vi "Dashboard Main.vi"() -> ()   [LabVIEW 2016]
uses:
  <vilib>/Rock Robotics/WPI/Dashboard/WPI_DashboardLogging Global.vi
  Robot Code/Common Code/Intake Status Cluster.ctl
  Robot Code/Common Code/Climb Status Cluster.ctl
  Robot Code/Common Code/Dash Display Data.ctl
  Robot Code/Common Code/Intake Commands.ctl
  Robot Code/Common Code/Intake Mode.ctl
  Robot Code/Common Code/Intake Presets.ctl
  Robot Code/Common Code/Dashboard Control Data.ctl
  Robot Code/Common Code/Drivetrain Presets.ctl
panel:
  in  "Rec Mode":enum32{"Stop", "Record", "Playback"}(radio)
  in  "Dashboard Tab":T1(tab)
  in  "DB Camera Config":bool
  out "Mbps LED":bool
  out "Mbps":dbl format="%#.1g"
  out "fps":dbl format="%#.1g"
  out "Camera Image":T2(plugin-control)
  out "Intake Power":dbl
  in  "Intake Presets":T3
  out "Intake Status Cluster":T4
  out "DS TCP":T7
  out "Robot Metrics":T8
  out "Camera Info":cluster{}
  in  "Camera Settings":T9={"Frame Rate"=30, "Compression"=30, "Size"=1} {"Frame Rate" scale=1.0..30.0; "Compression" scale=100.0..-1.0; "Size" items=["640x480", "320x240", "160x120"]}
  in  "TCP":refnum<k5>
  out "Robot IP":string
  in  "Camera Name":string(combo)="No Camera Selection"
  # "HW"
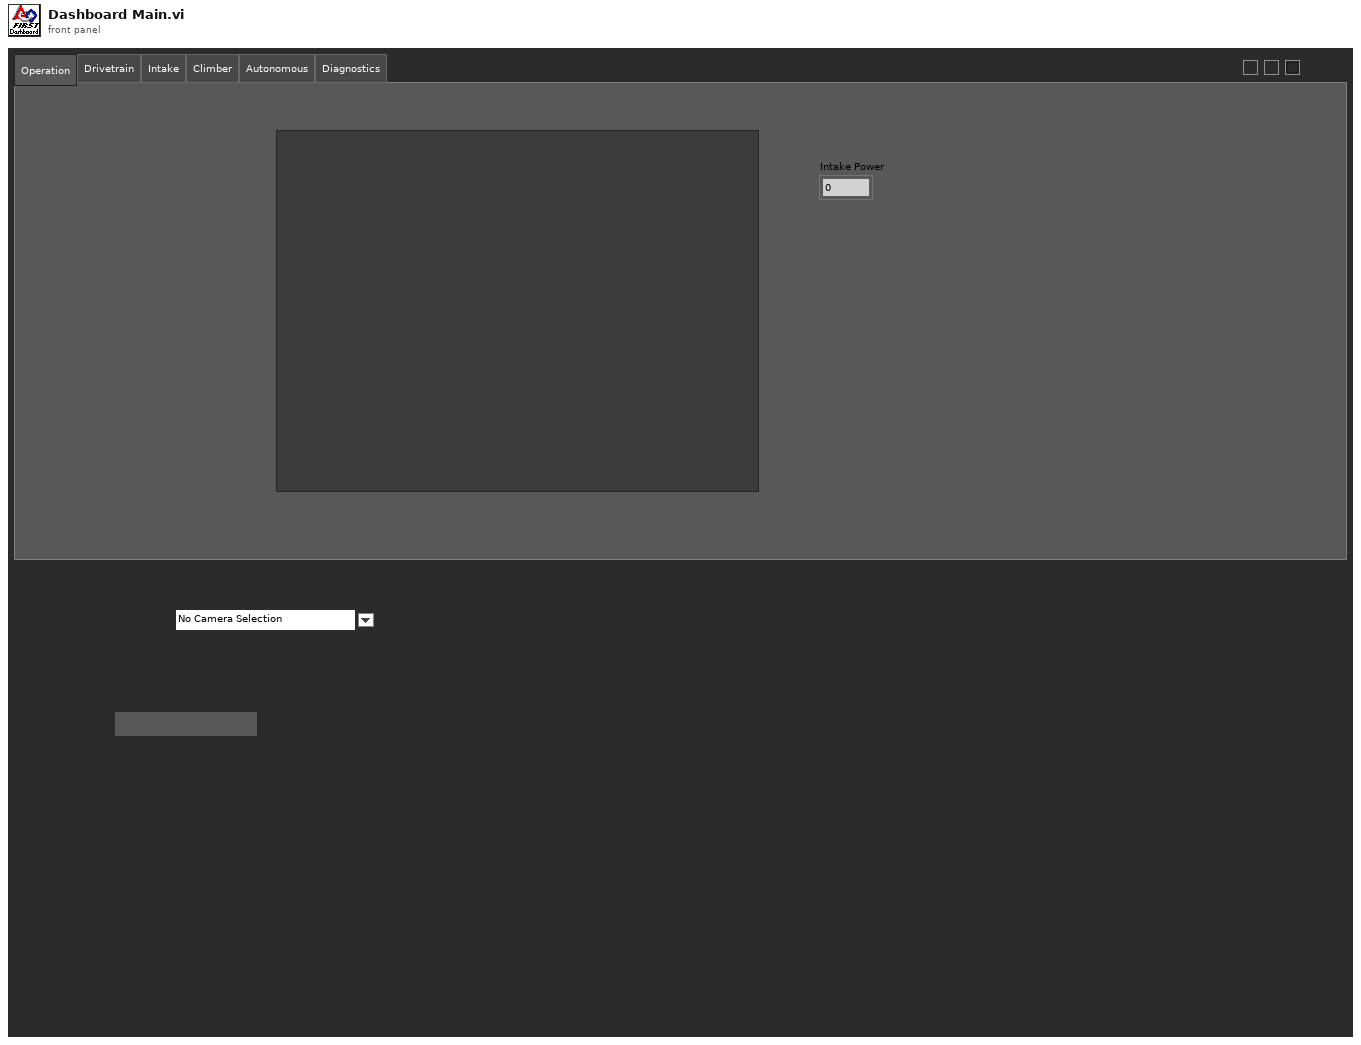
[diagram p1: front panel]
types:
  T1 = enum32{"Operation", "Drivetrain", "Intake", "Climber", "Autonomous", "Diagnostics"}
  T2 = typedef "IMAQ Image.ctl" = refnum<image>
  T3 = typedef "Intake Presets.ctl" = cluster{"Intake Power":dbl, "Outtake Power":dbl}
  T4 = typedef "Intake Status Cluster.ctl" = cluster{"Intake Power":dbl, "Intake Mode":T5, "Intake Command":T6}
  T5 = typedef "Intake Mode.ctl" = enum16{"Manual", "Auto"}
  T6 = typedef "Intake Commands.ctl" = enum16{"Idle", "Intake", "Outtake"}
  T7 = cluster{"Error Strings":string, "Disable Counts":cluster{u16, u16}, "Rail Faults":cluster{u16, u16, u16}, "Robot IP":string, "DB Mode":u8, "Event Info":cluster{"Name":string, "Type":u8, "Number":u16, "Replay":u8}, "Camera Addr":string}
  T8 = cluster{"Storage":cluster{"Disk Free":u64, "RAM Block":u32, "RAM free":u32}, "CPU Utilization":cluster{"CPU % ISR":sgl, "CPU % Time Crit":sgl, "CPU % Timed Str":sgl, "CPU % High":sgl, "CPU % Above":sgl, "CPU % Normal":sgl, "CPU % Low":sgl}, "CAN":cluster{"% Bus Utilization":sgl, "Bus Off Cnt":u32, "TX_FIFO Full Cnt":u32, "Receive Error Cnt":u8, "Transmit Error Cnt":u8}, "HID":cluster{"HID Outputs":u32, "Rumble Low":u16, "Rumble High":u16}[]}
  T9 = cluster{"Frame Rate":i32, "Compression":i32, "Size":u16}
  T10 = cluster{"IDs":cluster{"RPC field ID":u16, "Unique ID":u16}, "String":string}
  T11 = enum32{"Drive", "Basic", "Custom", "Test", "Checklist", "Variables"}
  T12 = typedef "Image Type" = u32
  T13 = typedef "Dashboard Control Data.ctl" = cluster{"Intake Presets":T3, "Drivetrain Presets":T14}
  T14 = typedef "Drivetrain Presets.ctl" = cluster{"Steer PID output":cluster{"output high":dbl, "output low":dbl}, " Steer PID gains":cluster{"proportional gain (Kc)":dbl, "integral time (Ti, min)":dbl, "derivative time (Td, min)":dbl}, "Gyro Tolerance":dbl}
  T15 = typedef "Dash Display Data.ctl" = cluster{"Intake Status Cluster ":T4, "Climb Status Cluster":T16}
  T16 = typedef "Climb Status Cluster.ctl" = cluster{"Power":dbl}
  T17 = cluster{"Status bits":cluster{"Test Mode":bool, "Autonomous":bool, "Enabled":bool, "Code Start":bool, "Brownout":bool, "Reserved 2":bool, "Reserved 3":bool, "E-Stop":bool}, "Code Trace":cluster{"Disabled":bool, "TeleOp":bool, "Auto":bool, "Test":bool}, "Controller Type":enum16{"unknown", "cRIO", "roboRio"}, "Code?":enum16{"unknown", "noCode", "code"}, "Battery V":dbl}
  T18 = cluster{"Control Bits":cluster{"TestMode":bool, "Autonomous":bool, "Enabled":bool, "FMS Present":bool, bool, bool, bool, "E-Stop":bool}, "Team Station ":u8, "Countdown":sgl, "Joystick Values":cluster{"Axes":dbl[], "Buttons":bool[], "POVs":i16[]}[]}
  T19 = enum8{"Tele-Op Disabled", "Tele-Op Enabled", "Auto Disabled", "Auto Enabled", "Test Disabled", "Test Enabled", "Disconnected", "No Code", "E-Stop"}
  T20 = cluster{"Image Size":bool, "Image Type":bool, "Pixel Value":bool, "ROI Information":bool, "Zoom Factor":bool}
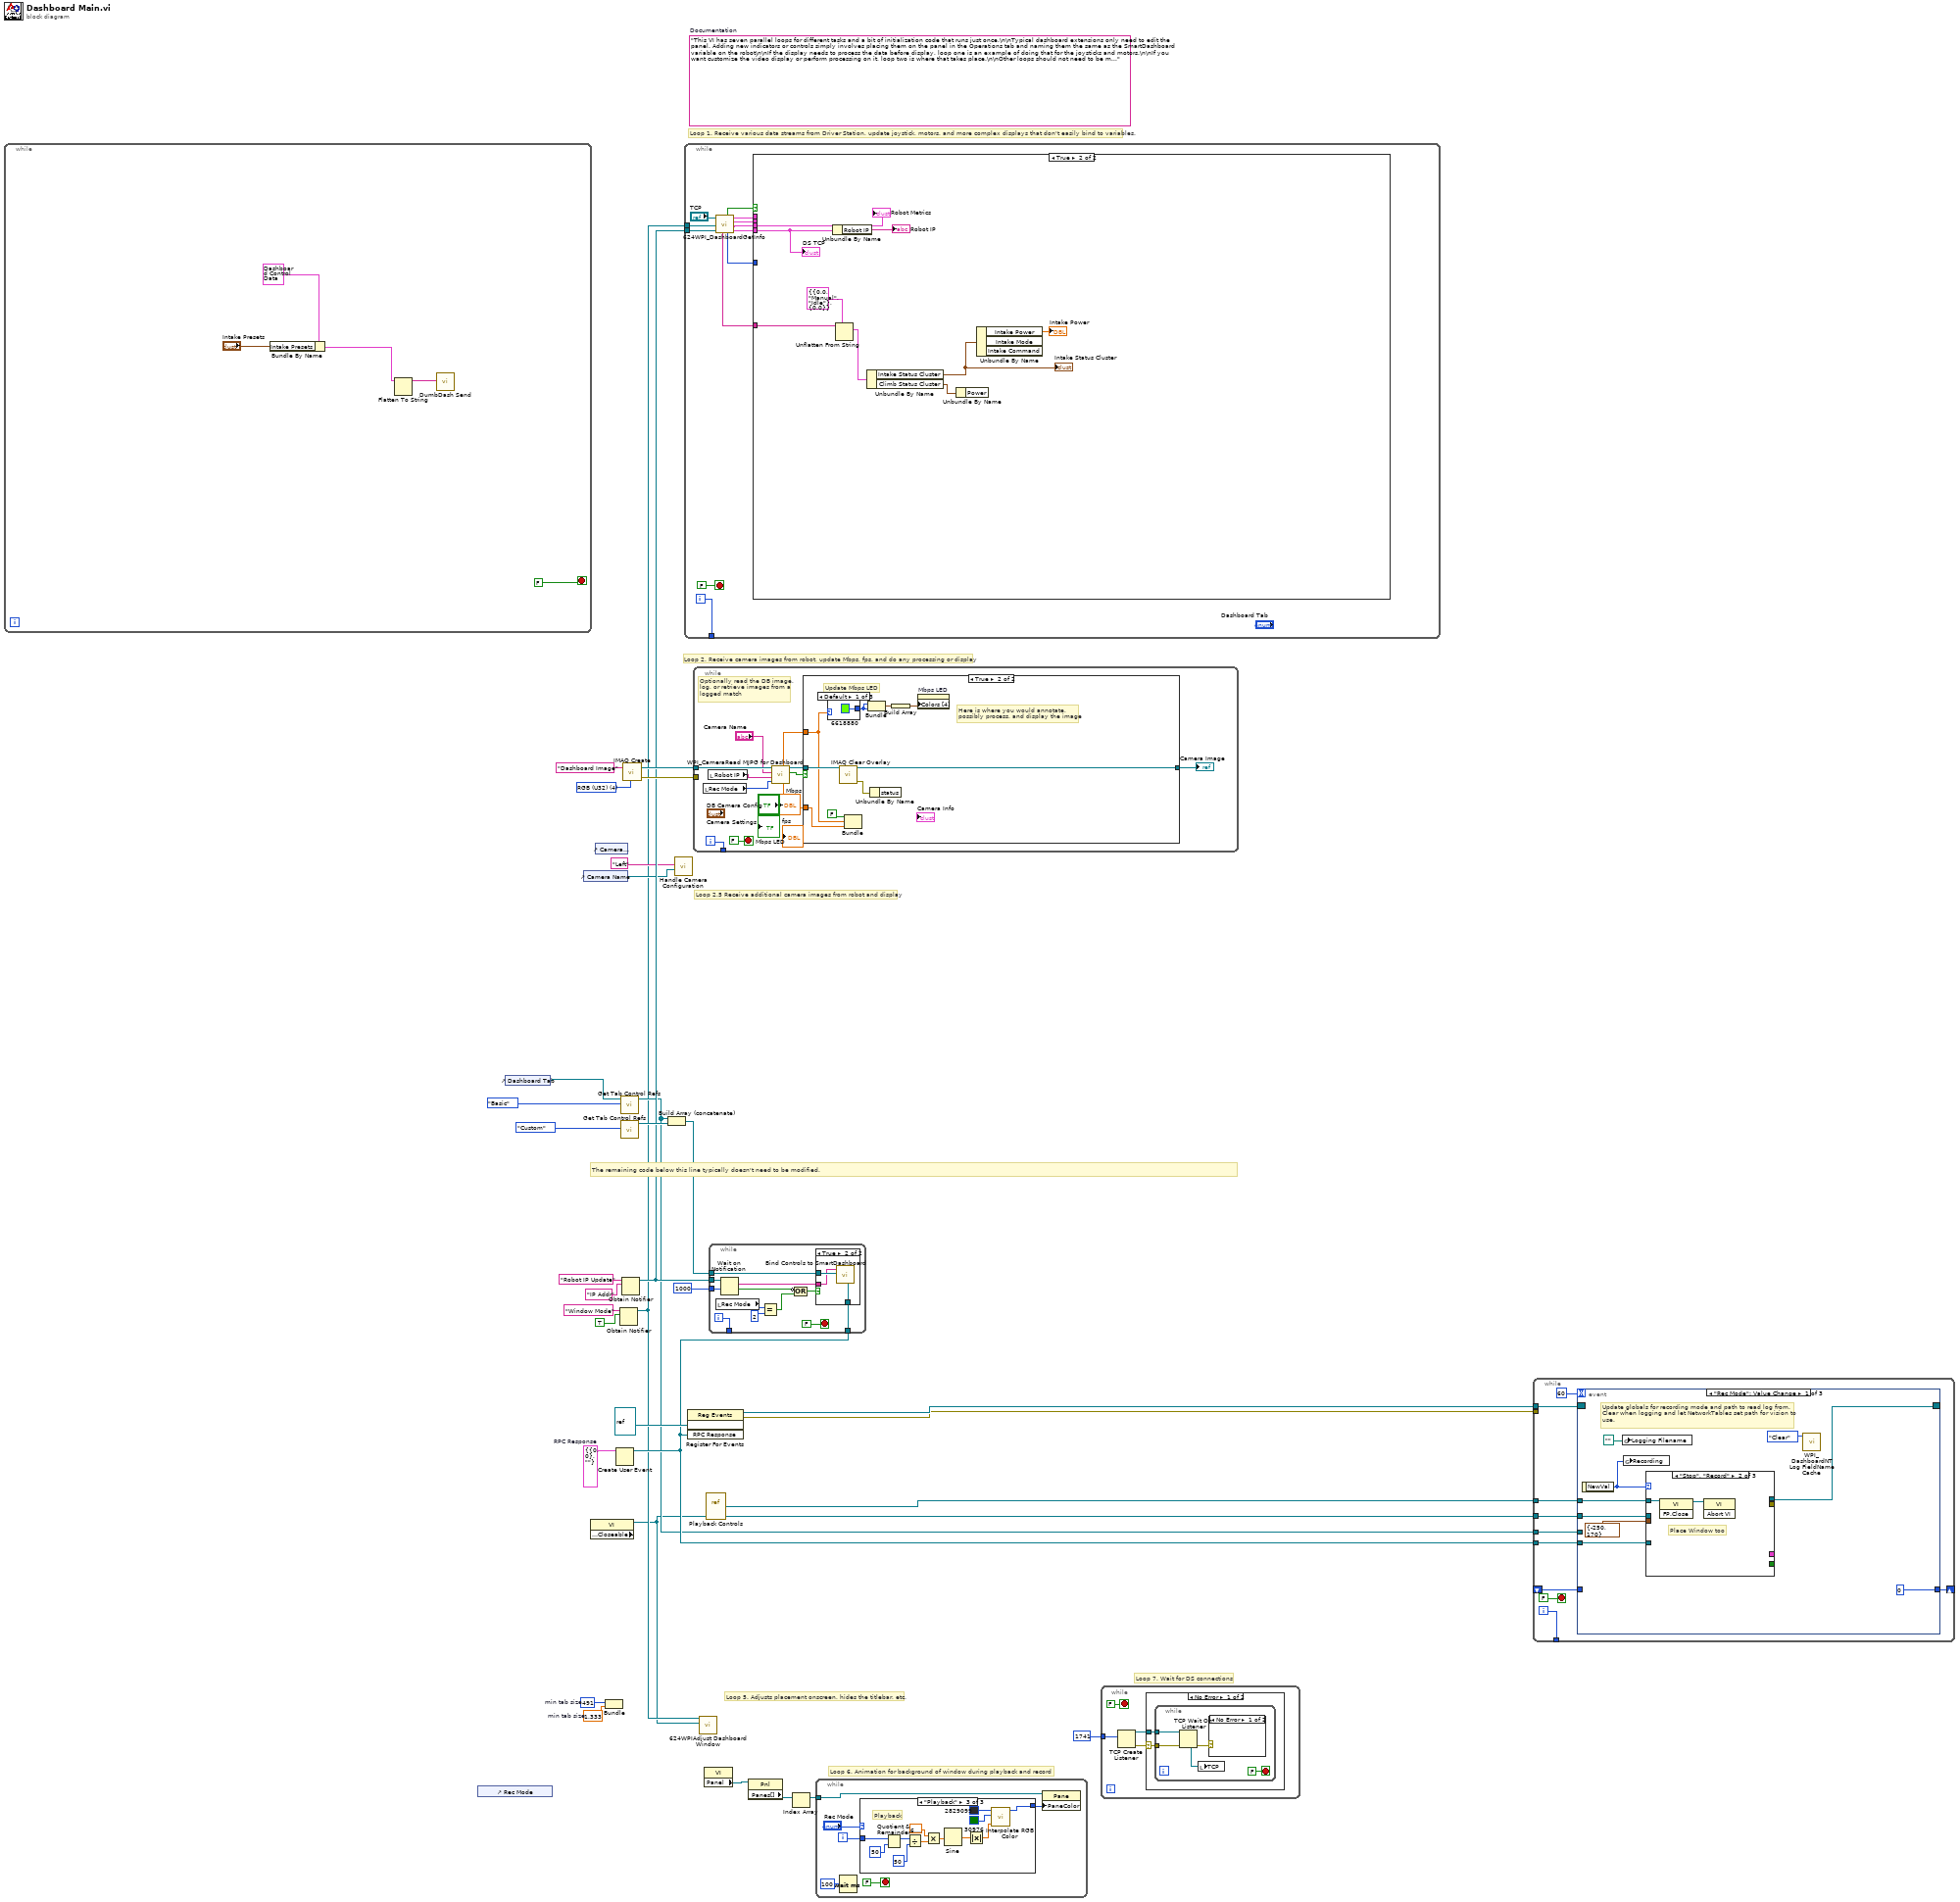
[diagram p0: block diagram]
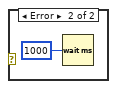
[diagram p2: hidden frame]
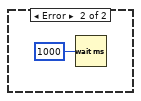
[diagram p3: hidden frame]
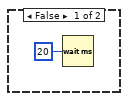
[diagram p4: hidden frame]
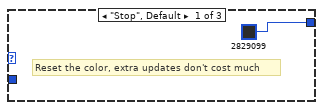
[diagram p5: hidden frame]
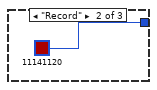
[diagram p6: hidden frame]
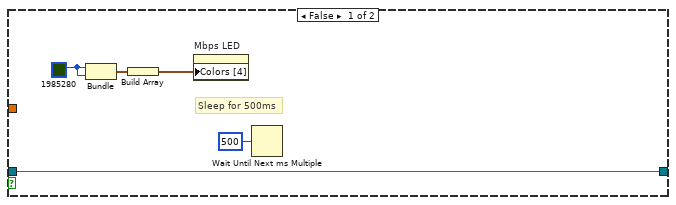
[diagram p8: hidden frame]
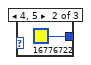
[diagram p9: hidden frame]
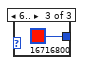
[diagram p10: hidden frame]
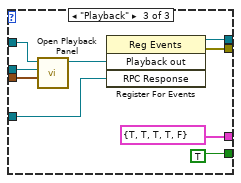
[diagram p12: hidden frame]
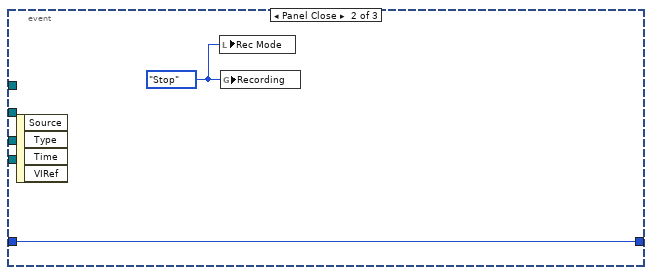
[diagram p13: hidden frame]
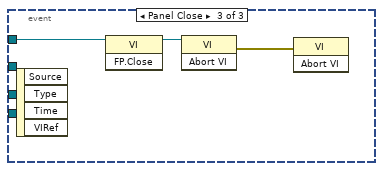
[diagram p14: hidden frame]
diagram:
  w8 = T10 {"IDs"={"RPC field ID"=0, "Unique ID"=0}, "String"=""}  # RPC Response
  w14 = 491  # min tab size
  w13 = 1.333  # min tab size
  (unwired) "This VI has seven parallel loops for different tasks and a bit of initialization code that runs just once.\n\nTypical dashboard extensions only need to edit the panel. Adding new indicators or controls simply involves placing them on the panel in the Operations tab and naming them the same as the SmartDashboard variable on the robot\n\nIf the display needs to process the data before display, loop one is an example of doing that for the joysticks and motors.\n\nIf you want customize the video display or perform processing on it, loop two is where that takes place.\n\nOther loops should not need to be modified. They are pretty standard, and document the task they perform."  # Documentation
  w32 = T12 4 items=["Grayscale (U8)", "Grayscale (I16)", "Grayscale (SGL)", "Complex (CSG)", "RGB (U32)", "HSL (U32)", "RGB (U64)"] ("Image Type")
  # "Loop 2.5 Receive additional camera images from robot and display"
  # "Loop 7. Wait for DS connections"
  # "Loop 6. Animation for background of window during playback and record"
  # "The remaining code below this line typically doesn't need to be modified."
  # "Loop 5. Adjusts placement onscreen, hides the titlebar, etc."
  # "Loop 1. Receive various data streams from Driver Station, update joystick, motors, and more complex displays that don't easily bind to variables."
  # "Loop 2. Receive camera images from robot, update Mbps, fps, and do any processing or display"
  n1 = while {
    stop <- FALSE stop-if-true
    n2 = Bundle By Name(cluster=T13 {"Intake Presets"={"Intake Power"=0.0, "Outtake Power"=0.0}, "Drivetrain Presets"={"Steer PID output"={"output high"=0.0, "output low"=0.0}, " Steer PID gains"={"proportional gain (Kc)"=0.0, "integral time (Ti, min)"=0.0, "derivative time (Td, min)"=0.0}, "Gyro Tolerance"=0.0}} ("Dashboard Packet"), "Intake Presets"="Intake Presets") -> (w34:T13)
    n3 = Flatten To String(anything=w34) -> (data string=w36:string)  [unwired: 3 in, 2 out]
    n4 = call "DumbDash Send.vi"("data string"=w36) -> ()  [unwired: 11 in]
  }
  n5 = control-ref of="Rec Mode"() -> ()  [unwired: 1 out]
  n6 = control-ref of="Dashboard Tab"() -> (w1:refnum<vi>)
  n7 = control-ref of="Camera Name"() -> (w6:refnum<vi>)
  n8 = property class="VI" props=["Front Panel.Closeable"]() -> (reference out=w2:refnum<vi>)  [unwired: 2 in, 2 out]
  n9 = control-ref of="Camera Settings"() -> ()  [unwired: 1 out]
  n10 = Bundle("min tab size"=w14, "min tab size"=w13) -> ()  [unwired: 1 in, 1 out]
  n11 = Create User Event(user event datatype=w8) -> (user event=w7:refnum<user-event>)  [unwired: 1 in, 1 out]
  n12 = Obtain Notifier(name (unnamed)="Window Mode", notification data type=TRUE) -> (notifier out=w3:refnum<notifier>)  [unwired: 2 in, 2 out]
  n13 = call <vilib>:"Get Tab Control Refs.vi"("Page Index"=T11."Basic" ("Dashboard Tab"), "TabControl in"=w1) -> ("ControlsOnPage"=w5:refnum<vi>[])  [unwired: 9 in]
  n14 = call <vilib>:"Get Tab Control Refs.vi"("Page Index"=T11."Custom" ("Dashboard Tab")) -> ("ControlsOnPage"=w16:refnum<vi>[])  [unwired: 10 in]
  n15 = Obtain Notifier(name (unnamed)="Robot IP Update", notification data type="IP Addr" ("name (unnamed)")) -> (notifier out=w10:refnum<notifier>)  [unwired: 2 in, 2 out]
  n16 = call "IMAQ Create"("Image Name"="Dashboard Image", "Image Type"=w32) -> ("New Image"=w30:T2, "error out"=w29:errorcluster)  [unwired: 2 in, 1 out]
  n17 = Build Array (concatenate)(w5, w16) -> (w15:refnum<vi>[])
  n18 = call "Handle Camera Configuration.vi"("CameraNameRef"=w6, "Camera File Name"="Left") -> ()  [unwired: 10 in]
  n19 = while {
    tunnel: [w48] -> _
    tunnel: w10 -> [w39]
    tunnel: w3 -> [w40]
    i -> [w48]
    stop <- FALSE stop-if-true
    n20 = call "624WPI_DashboardGetInfo.vi"("Binding Refnum"=w39, "Window Mode Notifier"=w40, "TCP Cnx"="TCP") -> ("Power and Errors"=w44:T7, "Robot Metrics"=w45:T8, "Status Info"=w46:T17, "Control Info"=w47:T18, "Robot Mode"=w43:T19, "Process?"=w42:bool, "Custom Dashboard Data"=w38:string)  [unwired: 2 in]
    n21 = case shown="True" w42 {
      tunnel: w46 -> [_ _]
      tunnel: w45 -> [_ w57]
      tunnel: w47 -> [_ _]
      tunnel: w44 -> [_ w59]
      tunnel: w43 -> [_ _]
      tunnel: w38 -> [_ w56]
      frame False {
        n22 = Wait (ms)(milliseconds to wait=u32 20) -> ()  [unwired: 1 out]
      }
      frame True {
        n23 = Unbundle By Name(w59) -> ("Robot IP"=→"Robot IP":string)
        n24 = Unflatten From String(type=T15 {"Intake Status Cluster "={"Intake Power"=0.0, "Intake Mode"=enum."Manual", "Intake Command"=enum."Idle"}, "Climb Status Cluster"={"Power"=0.0}} ("Dashboard Display Data"), binary string=w56) -> (value=w54:T15)  [unwired: 3 in, 2 out]
        n25 = Unbundle By Name(w54) -> ("Intake Status Cluster"=w53:T4, "Climb Status Cluster"=w52:T16)
        "Intake Status Cluster" <- w53
        n26 = Unbundle By Name(w52) -> ()  [unwired: 1 out]
        n27 = Unbundle By Name(w53) -> ("Intake Power"=→"Intake Power":dbl)  [unwired: 2 out]
        "DS TCP" <- w59
        "Robot Metrics" <- w57
      }
    }
  }
  n28 = register-events(refnum<vi> refnum, w7) -> (reference out=w20:refnum<event-registration>, error out=w19:errorcluster)  [unwired: 2 in]
  n29 = while {
    tunnel: w30 -> [w68]
    tunnel: w29 -> [_]
    tunnel: [w69] -> _
    i -> [w69]
    stop <- FALSE stop-if-true
    # "Optionally read the DB image,\nlog, or retrieve images from a\nlogged match"
    n30 = local read "Rec Mode"() -> (w64:enum32{"Stop", "Record", "Playback"})
    n31 = local read "Robot IP"() -> (w63:string)
    n32 = call <vilib>:"WPI_CameraRead MJPG for Dashboard.vi"("Rec Mode"=w64, "Robot IP"=w63, "Camera Name"="Camera Name", "Refnum in"=w68) -> ("Active"=w66:bool, "Refnum out"=w67:T2, "FPS"=w65:dbl, "Bandwidth (Mbps)"=w62:dbl)  [unwired: 4 in]
    n33 = case shown="True" w66 {
      tunnel: w67 -> [w71 w81]
      tunnel: w62 -> [_ w78]
      tunnel: w65 -> [_ w79]
      tunnel: [w71 w76] -> w60
      frame False {
        w73 = u32 1985280 ("Color Box")
        # "Sleep for 500ms"
        n34 = Bundle("Color Box"=w73, "Color Box"=w73) -> (w74:cluster{"Color Box":u32, "Color Box":u32})  [unwired: 1 out]
        n35 = Build Array(w74) -> (w72:cluster{"Color Box":u32, "Color Box":u32}[])
        n36 = property on="Mbps LED" class="Bool (strict)"("Colors [4]"=w72) -> ()  [unwired: 2 in, 2 out]
        n37 = Wait Until Next ms Multiple(millisecond multiple=u32 500) -> ()  [unwired: 1 out]
      }
      frame True {
        # "Here is where you would annotate,\npossibly process, and display the image"
        # "Update Mbps LED"
        n38 = case shown="Default" w78 {
          tunnel: [u32 6618880 ("Color Box") u32 16776722 ("Color Box") u32 16716800 ("Color Box")] -> w82
          frame Default {
          }
          frame 4, 5 {
          }
          frame 6.. {
          }
        }
        n39 = call "IMAQ Clear Overlay"("Image"=w81) -> ("error out"=w84:errorcluster, "Image Out"=w76:T2)  [unwired: 2 in, 7 out]
        n40 = Bundle(FALSE, "Bandwidth (Mbps)"=w78, "FPS"=w79) -> ()  [unwired: 1 in, 1 out]
        n41 = Bundle("Color Box"=w82, "Color Box"=w82) -> (w83:cluster{"Color Box":u32, "Color Box":u32})  [unwired: 1 out]
        n42 = Unbundle By Name(w84) -> ()  [unwired: 1 out]
        n43 = Build Array(w83) -> (w80:cluster{"Color Box":u32, "Color Box":u32}[])
        n44 = property on="Mbps LED" class="Bool (strict)"("Colors [4]"=w80) -> ()  [unwired: 2 in, 2 out]
      }
    }
    "Camera Image" <- w60
  }
  n45 = call "624WPIAdjust Dashboard Window.vi"("VI"=w2, "Notifier in"=w3) -> ()  [unwired: 10 in]
  n46 = property class="VI"() -> ("Panel"=w23:refnum<vi>)  [unwired: 2 in, 2 out]
  n47 = vi-ref "Playback Controls.vi"() -> (w21:refnum<vi>)
  n48 = while {
    tunnel: w15 -> [w99]
    tunnel: w10 -> [w97]
    tunnel: [w95] -> _
    tunnel: u32 1000 ("milliseconds to wait") -> [w94]
    tunnel: w7 -> [w88]
    i -> [w95]
    stop <- FALSE stop-if-true
    n49 = local read "Rec Mode"() -> (w90:enum32{"Stop", "Record", "Playback"})
    n50 = Wait on Notification(notifier=w97, timeout in ms (-1)=w94) -> (notification=w96:string, timed out?=w92:bool)  [unwired: 2 in, 2 out]
    n51 = Equal?(x=w90, y=u16 2 ("Rec Mode")) -> (x = y?=w91:bool)
    n52 = Compound Arithmetic op=OR(invert w92, w91) -> (w93:bool)
    n53 = case shown="True" w93 {
      tunnel: w99 -> [_ w102]
      tunnel: w96 -> [_ w101]
      tunnel: w88 -> [_ w100]
      frame False {
      }
      frame True {
        n54 = call <vilib>:"Bind Controls to SmartDashboard.vi"("RPC ref"=w100, "Bound Control Refs"=w102, "Server IP Address"=w101) -> ()  [unwired: 9 in]
      }
    }
  }
  n55 = property class="Pnl"(reference=w23) -> ("Panes[]"=w24:refnum<vi>[])  [unwired: 1 in, 2 out]
  n56 = Index Array(array=w24) -> (element=w22:refnum<vi>)  [unwired: 1 in]
  n57 = while {
    tunnel: w22 -> [w104]
    i -> [w107]
    stop <- FALSE stop-if-true
    n58 = Wait (ms)(milliseconds to wait=u32 100) -> ()  [unwired: 1 out]
    n59 = case shown="\"Playback\"" "Rec Mode" {
      tunnel: w107 -> [_ _ w122]
      tunnel: [u32 2829099 ("Base Color") u32 11141120 ("Target Color") w111] -> w103
      frame "Stop", Default {
        # "Reset the color, extra updates don't cost much"
      }
      frame "Record" {
      }
      frame "Playback" {
        # "Playback"
        n60 = Quotient & Remainder(x=w122, y=u32 50 ("milliseconds to wait")) -> (x-y*floor(x/y)=w118:u32)  [unwired: 1 out]
        n61 = Divide(x=w118, y=u32 50 ("milliseconds to wait")) -> (x/y=w115:dbl)
        n62 = Multiply(x=6.283185307179586, y=w115) -> (x*y=w120:dbl)
        n63 = Sine(x=w120) -> (sin(x)=w119:dbl)
        n64 = Absolute Value(x=w119) -> (abs(x)=w112:dbl)
        n65 = call "Interpolate RGB Color.vi"("Proportion"=w112, "Target Color"=u32 30976, "Base Color"=u32 2829099) -> ("Result Color"=w111:u32)  [unwired: 8 in]
      }
    }
    n66 = property class="Pane"(reference=w104, "PaneColor"=w103) -> ()  [unwired: 1 in, 2 out]
  }
  n67 = while {
    tunnel: u16 1741 ("timeout ms (25000)") -> [w124]
    stop <- FALSE stop-if-true
    n68 = TCP Create Listener(10:w124) -> (0:w123:errorcluster, 3:w125:refnum<k5>)  [unwired: 4 in, 1 out]
    n69 = case shown="No Error" w123 {
      selector: w123 -> [w127 _]
      tunnel: w125 -> [w128 _]
      frame No Error {
        n70 = while {
          tunnel: w128 -> [w131]
          tunnel: w127 -> [w130]
          stop <- FALSE stop-if-true
          n71 = TCP Wait On Listener(8:w130, 11:w131) -> (0:w132:errorcluster, 4:w133:refnum<k5>)  [unwired: 2 in, 3 out]
          n72 = local write "TCP"(w133) -> ()
          n73 = case shown="No Error" w132 {
            frame No Error {
            }
            frame Error {
              n74 = Wait (ms)(milliseconds to wait=u32 1000) -> ()  [unwired: 1 out]
            }
          }
        }
      }
      frame Error {
        n75 = Wait (ms)(milliseconds to wait=u32 1000) -> ()  [unwired: 1 out]
      }
    }
  }
  n76 = while {
    tunnel: [w143] -> _
    tunnel: w21 -> [w142]
    tunnel: w20 -> [w141]
    tunnel: w19 -> [_]
    tunnel: w2 -> [w140]
    tunnel: w7 -> [w139]
    shift-right: [w138] -> _
    shift-left: _ -> [w137]
    tunnel: w5 -> [w136]
    i -> [w143]
    stop <- FALSE stop-if-true
    n77 = event shown="[0] \"Rec Mode\": Value Change" {
      selector: w141 -> [_ _ _]
      dyn-events: [w151 _ _] -> _
      timeout: u32 60 ("milliseconds to wait") -> [_ _ _]
      tunnel: w142 -> [w153 _ w170]
      tunnel: w140 -> [w149 _ _]
      tunnel: w139 -> [w147 _ _]
      tunnel: [0 w166 _] -> w138
      tunnel: w137 -> [_ w166 _]
      tunnel: w136 -> [_ _ _]
      event "Rec Mode": Value Change {
        # "Update globals for recording mode and path to read log from.\nClear when logging and let NetworkTables set path for vision to\nuse."
        n78 = event-data() -> ("NewVal"=w154:enum32{"Stop", "Record", "Playback"})  [unwired: 1 in]
        n79 = global write "WPI_DashboardLogging Global.vi" "Logging Filename"(path "") -> ()
        n80 = global write "WPI_DashboardLogging Global.vi" "Recording"(w154) -> ()
        n81 = case shown="\"Stop\", \"Record\"" w154 {
          tunnel: w153 -> [_ w156 w165]
          tunnel: [_ _ w164] -> w151
          tunnel: [_ _ w163] -> _
          tunnel: w149 -> [_ _ w161]
          tunnel: cluster{i32, i32} {-250, 170} -> [_ _ w160]
          tunnel: [_ _ T20 {"Image Size"=TRUE, "Image Type"=TRUE, "Pixel Value"=TRUE, "ROI Information"=TRUE, "Zoom Factor"=FALSE} ("Image Information Shown:All Elements")] -> _
          tunnel: [_ _ TRUE ("Zoom Factor")] -> _
          tunnel: w147 -> [_ _ w157]
          frame Default {
          }
          frame "Stop", "Record" {
            # "Place Window too"
            n82 = invoke class="VI" method="FP.Close"(reference=w156) -> (reference out=w155:refnum<vi>)  [unwired: 2 in, 2 out]
            n83 = invoke class="VI" method="Abort VI"(reference=w155) -> ()  [unwired: 2 in, 3 out]
          }
          frame "Playback" {
            n84 = call "Open Playback Panel.vi"("Offset"=w160, "DB VI Ref"=w161, "Playback in"=w165) -> ("Playback out"=w162:refnum<vi>)  [unwired: 8 in]
            n85 = register-events(w162, w157) -> (reference out=w164:refnum<event-registration>, error out=w163:errorcluster)  [unwired: 2 in]
          }
        }
        n86 = call <vilib>:"WPI_DashboardNT Log FieldName Cache.vi"("Operation"=enum16{"Lookup/Add", "Index", "Clear"}."Clear") -> ()  [unwired: 8 in, 3 out]
      }
      event Panel Close {
        w167 = enum32{"Stop", "Record", "Playback"}."Stop" ("Rec Mode")
        n87 = event-data() -> ()  [unwired: 1 in, 4 out]
        n88 = local write "Rec Mode"(w167) -> ()
        n89 = global write "WPI_DashboardLogging Global.vi" "Recording"(w167) -> ()
      }
      event Panel Close {
        n90 = event-data() -> ()  [unwired: 1 in, 4 out]
        n91 = invoke class="VI" method="FP.Close"(reference=w170) -> (reference out=w169:refnum<vi>)  [unwired: 2 in, 2 out]
        n92 = invoke class="VI" method="Abort VI"(reference=w169) -> (error out=w168:errorcluster)  [unwired: 2 in, 2 out]
        n93 = invoke class="VI" method="Abort VI"(error in=w168) -> ()  [unwired: 2 in, 3 out]
      }
    }
  }
